vi "move.vi"(8 "error in (no error)":errorcluster, 9 "y":i32, 10 "x":i32, 11 "CompoundShape in":refnum<class "CompoundShape.lvclass">) -> (0 "error out":errorcluster, 3 "CompoundShape out":refnum<class "CompoundShape.lvclass">)   [LabVIEW 2018, in "CompoundShape.lvclass"]
uses:
  CompoundShape.lvclass
  Shape Class/Shape.lvclass
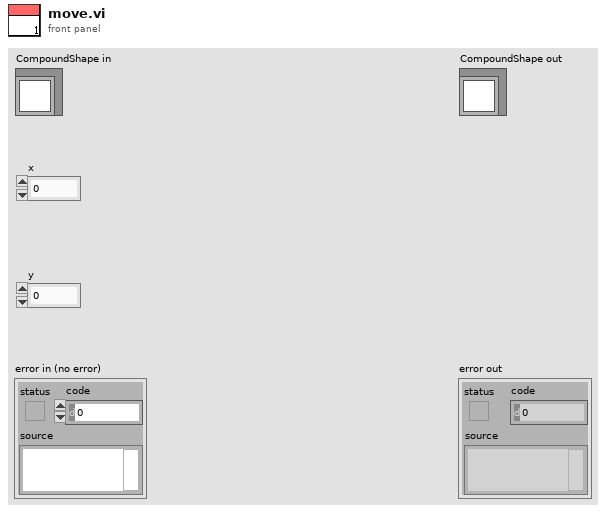
[diagram p1: front panel]
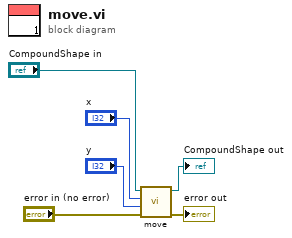
[diagram p0: block diagram]
diagram:
  n1 = call-parent "move.vi"("error in (no error)"="error in (no error)", "y"="y", "x"="x", "Shape in"="CompoundShape in") -> ("error out"=→"error out":errorcluster, "Shape out"=→"CompoundShape out":refnum<class "CompoundShape.lvclass">)  [unwired: 6 in]
